vi "Send Launch Nested Panel Message.vi"(4 "Auto-stop? (T)":bool=TRUE, 6 "timeout in ms (-1)":i32=-1, 7 "Priority":T1=enum."Normal" caption="Message Priority (Normal)", 8 "error in (no error)":errorcluster, 9 "Panel":refnum<class "Panel.lvclass">, 10 "Nested Panel Actor":refnum<class "Panel Actor.lvclass">, 11 "Message Enqueuer in":refnum<class "Message Enqueuer.lvclass">) -> (0 "error out":errorcluster, 1 "timed out?":bool, 2 "Nested Actor's Q":refnum<class "Message Enqueuer.lvclass">)   [LabVIEW 2017, in "MGI-Panel Actor.lvlib" / "Launch Nested Panel Message Msg.lvclass"]
doc: "Sends the <b>Launch Nested Panel Message Msg.lvclass</b> message.\n\nThis message will call <b>Launch Nested Panel Message.vi</b> on the <b>MGI-Panel Actor.lvlib:Panel Actor.lvclass</b> actor.\n\n<b>Launch Nested Panel Message.vi Description</b>\nAccess scope wrapper to the private message can send a launch nested panel message.\n\n----\nPlease see the following web address for additional documentation and tutorial information:\nhttp://www.mooregoodideas.com/mgi-panel-manager/\n\nAuthor: Derek Trepanier\n\nCopyright (c) 2018, Moore Good Ideas, Inc.\n\nAll rights reserved.\n\nRedistribution and use in source and binary forms, with or without modification, are permitted provided that the following conditions are met:\n\n * Redistributions of source code must retain the above copyright notice, this list of conditions and the following disclaimer.\n * Redistributions in binary form must reproduce the above copyright notice, this list of conditions and the following disclaimer in the documentation and/or other materials provided with the distribution.\n * Neither the name of Moore Good Ideas, Inc. nor the names of its contributors may be used to endorse or promote products derived from this software without specific prior written permission.\n\nTHIS SOFTWARE IS PROVIDED BY THE COPYRIGHT HOLDERS AND CONTRIBUTORS \"AS IS\" AND ANY EXPRESS OR IMPLIED WARRANTIES, INCLUDING, BUT NOT LIMITED TO, THE IMPLIED WARRANTIES OF MERCHANTABILITY AND FITNESS FOR A PARTICULAR PURPOSE ARE DISCLAIMED. IN NO EVENT SHALL THE COPYRIGHT OWNER OR CONTRIBUTORS BE LIABLE FOR ANY DIRECT, INDIRECT, INCIDENTAL, SPECIAL, EXEMPLARY, OR CONSEQUENTIAL DAMAGES (INCLUDING, BUT NOT LIMITED TO, PROCUREMENT OF SUBSTITUTE GOODS OR SERVICES; LOSS OF USE, DATA, OR PROFITS; OR BUSINESS INTERRUPTION) HOWEVER CAUSED AND ON ANY THEORY OF LIABILITY, WHETHER IN CONTRACT, STRICT LIABILITY, OR TORT (INCLUDING NEGLIGENCE OR OTHERWISE) ARISING IN ANY WAY OUT OF THE USE OF THIS SOFTWARE, EVEN IF ADVISED OF THE POSSIBILITY OF SUCH DAMAGE."
uses:
  Launch Nested Panel Message Msg.lvclass
  <vilib>/ActorFramework/Message Enqueuer/Message Enqueuer.lvclass
  <vilib>/ActorFramework/Message Enqueuer/Message Priority.ctl
  Panel Actor/Panel Actor.lvclass
  panel-manager/Source/Panel/Panel.lvclass
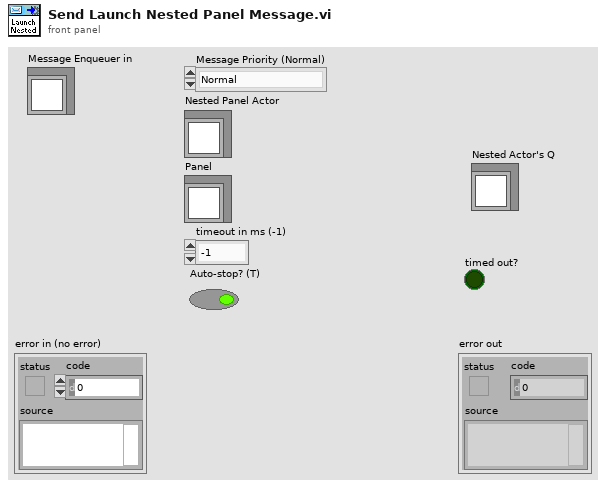
[diagram p1: front panel]
types:
  T1 = typedef "Actor Framework.lvlib/Message Enqueuer.lvclass/Message Priority.ctl" = enum16{"Low", "Normal", "High"}
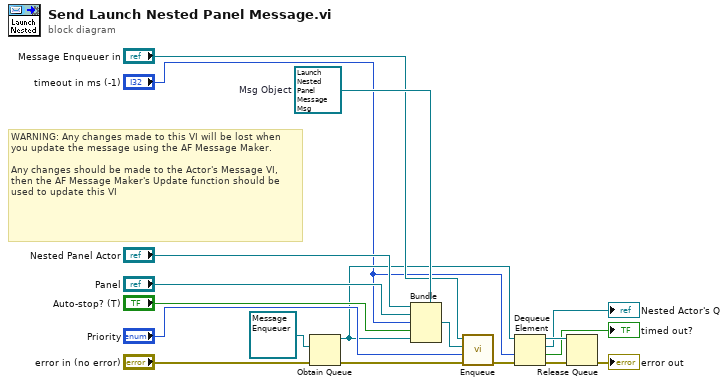
[diagram p0: block diagram]
diagram:
  w15 = refnum<class "Launch Nested Panel Message Msg.lvclass"> refnum  # Msg Object
  # "WARNING: Any changes made to this VI will be lost when you update the message using the AF Message Maker.\n\nAny changes should be made to the Actor's Message VI, then the AF Message Maker's Update function should be used to update this VI"
  n1 = Obtain Queue(element data type=refnum<class "Message Enqueuer.lvclass"> refnum ("Message Enqueuer in"), error in (no error)="error in (no error)") -> (queue out=w8:refnum<queue>, error out=w9:errorcluster)  [unwired: 3 in, 1 out]
  n2 = Bundle(cluster=w15, "Nested Panel Actor", "Panel", "timeout in ms (-1)", "Auto-stop? (T)", w8) -> (w13:refnum<class "Launch Nested Panel Message Msg.lvclass">)
  n3 = call <vilib>:"Enqueue.vi"("error in (no error)"=w9, "Message Priority (Normal)"="Priority", "Message"=w13, "Message Enqueuer in"="Message Enqueuer in") -> ("error out"=w7:errorcluster)  [unwired: 6 in, 1 out]
  n4 = Dequeue Element(queue=w8, timeout in ms (-1)="timeout in ms (-1)", error in (no error)=w7) -> (queue out=w5:refnum<queue>, element=→"Nested Actor's Q":refnum<class "Message Enqueuer.lvclass">, timed out?=→"timed out?":bool, error out=w4:errorcluster)
  n5 = Release Queue(queue=w5, error in (no error)=w4) -> (error out=→"error out":errorcluster)  [unwired: 1 in, 2 out]
